vi "Connect PV.vi"(8 "error in (no error)":errorcluster, 10 "PV URL":string, 11 "CS++DSMonitor in":refnum<class "CS++DSMonitor.lvclass">) -> (0 "error out":errorcluster, 3 "CS++DSMonitor out":refnum<class "CS++DSMonitor.lvclass">)   [LabVIEW 2016, in "CS++DSMonitor.lvlib" / "CS++DSMonitor.lvclass"]
doc: "Open connection to process variable."
uses:
  CS++DSMonitor.lvclass
  CS++DSMonitor.lvclass/CS++DSMonitor.ctl
  Libraries/Utilities/CS++Utilities.lvlib
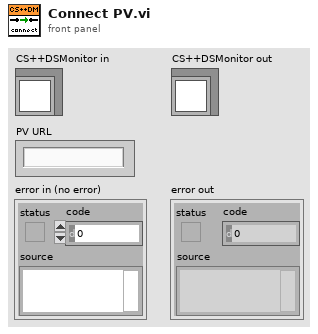
[diagram p1: front panel]
types:
  T1 = enum16{"Read", "Write", "ReadWrite", "BufferedRead", "BufferedReadWrite"}
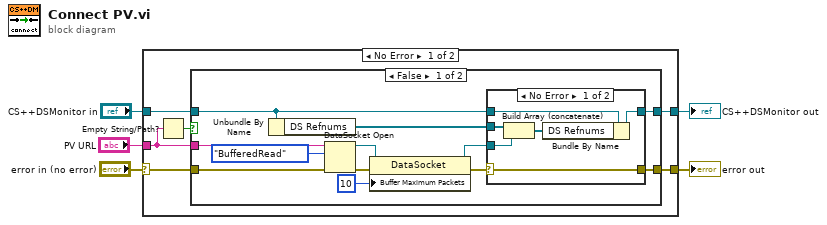
[diagram p0: block diagram]
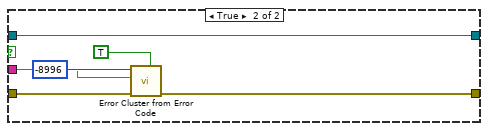
[diagram p3: hidden frame]
diagram:
  n1 = case shown="No Error" "error in (no error)" {
    selector: "error in (no error)" -> [w11 w39]
    tunnel: [w8 w39] -> w2
    tunnel: [w9 w38] -> w3
    tunnel: "CS++DSMonitor in" -> [w10 w38]
    tunnel: "PV URL" -> [w7 _]
    frame No Error {
      n2 = Empty String/Path?(string/path=w7) -> (empty?=w6:bool)
      n3 = case shown="False" w6 {
        tunnel: w11 -> [w17 w35]
        tunnel: w7 -> [w18 w32]
        tunnel: w10 -> [w23 w37]
        tunnel: [w22 w37] -> w9
        tunnel: [w20 w34] -> w8
        frame False {
          n4 = Unbundle By Name(w23) -> ("DS Refnums"=w21:refnum<k13>[])
          n5 = DataSocket Open(8:w17, 10:T1."BufferedRead" ("mode"), 11:w18) -> (0:w16:errorcluster, 3:w14:refnum<k13>)  [unwired: 1 in]
          n6 = property class="DataSocket"(reference=w14, error in=w16, "Buffer Maximum Packets"=10) -> (reference out=w13:refnum<k13>, error out=w15:errorcluster)
          n7 = case shown="No Error" w15 {
            selector: w15 -> [w24 w30]
            tunnel: w13 -> [w29 _]
            tunnel: w23 -> [w28 w31]
            tunnel: [w27 w31] -> w22
            tunnel: w21 -> [w25 _]
            tunnel: [w24 w30] -> w20
            frame No Error {
              n8 = Build Array (concatenate)(w25, w29) -> (w26:refnum<k13>[])
              n9 = Bundle By Name(cluster=w28, "DS Refnums"=w26) -> (w27:refnum<class "CS++DSMonitor.lvclass">)
            }
            frame Error {
            }
          }
        }
        frame True {
          n10 = call "Error Cluster from Error Code.vi"("is warning? (False)"=TRUE, "Error In"=w35, "Error Message (\"\")"=w32, "Error Code (0)"=-8996 ("error code (no error:0)")) -> ("Error Out"=w34:errorcluster)  [unwired: 7 in]
        }
      }
    }
    frame Error {
    }
  }
  "error out" <- w2
  "CS++DSMonitor out" <- w3
